vi "test_led_count1.vi"(9 "Reset":bool caption="重置", 10 "Time Target (s)":dbl caption="目标时间(s)", 11 "当前档位":string) -> (2 "输出文本":string, 3 "Time has Elapsed":bool caption="计时结束")   [LabVIEW 2016]
panel:
  out "子字符串;substring 2":string
  out "子字符串;substring":string
  out "Elapsed Time Text":string caption="已用时间文本"
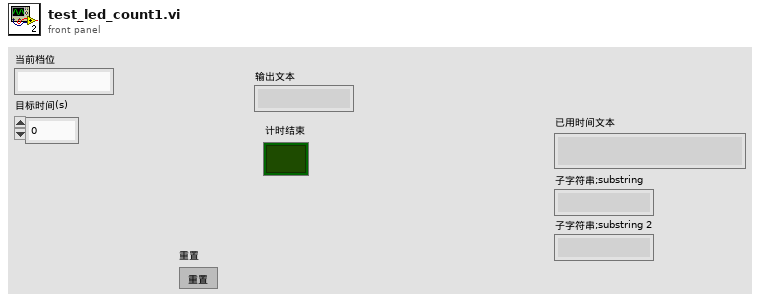
[diagram p1: front panel]
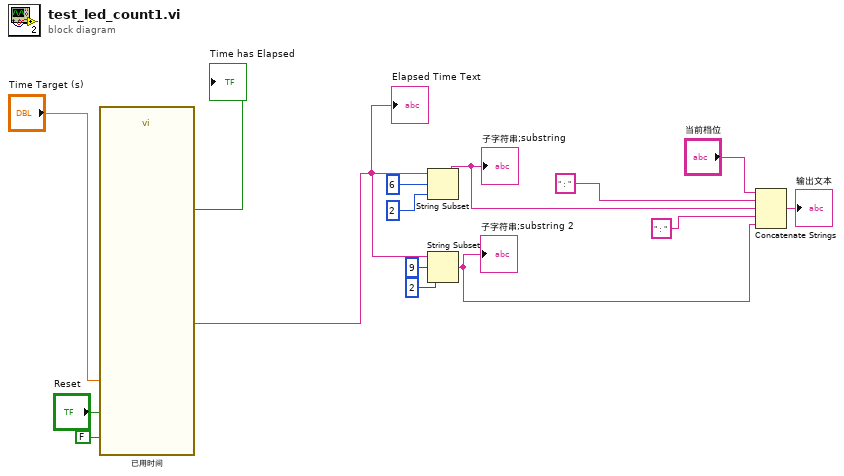
[diagram p0: block diagram]
diagram:
  n1 = call "已用时间"("Time Target (s)"="Time Target (s)", "Reset"="Reset", "Auto Reset"=FALSE) -> ("Time has Elapsed"=→"Time has Elapsed":bool, "Elapsed Time Text"=w13:string)  [unwired: 9 in, 6 out]
  "Elapsed Time Text" <- w13
  n2 = String Subset(string=w13, offset (0)=6 ("偏移量(0)"), length (rest)=2 ("长度（剩余）")) -> (substring=w8:string)
  "子字符串;substring" <- w8
  n3 = String Subset(string=w13, offset (0)=9 ("偏移量(0)"), length (rest)=2 ("长度（剩余）")) -> (substring=w9:string)
  "子字符串;substring 2" <- w9
  n4 = Concatenate Strings("当前档位", "：", w8, "：" ("字符串"), w9) -> (→"输出文本":string)
